vi "ROI selection.vi"(2 "ROI":T1={"Far Field  Row"=72, "Far Field Col"=185, "Far Field outer radius"=62, "Far Field inner radius"=62}, 3 "Far Field pixels":T2, 4 "Near Field pixels":T3) -> (0 "Far Field ROI":T2, 1 "Near Field ROI":T3)   [LabVIEW 2020]
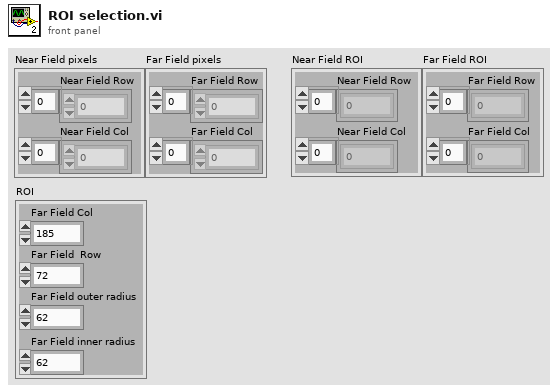
[diagram p1: front panel]
types:
  T1 = cluster{"Far Field  Row":i32, "Far Field Col":i32, "Far Field outer radius":i32, "Far Field inner radius":i32}
  T2 = cluster{"Far Field Row":dbl[], "Far Field Col":dbl[]}
  T3 = cluster{"Near Field Row":dbl[], "Near Field Col":dbl[]}
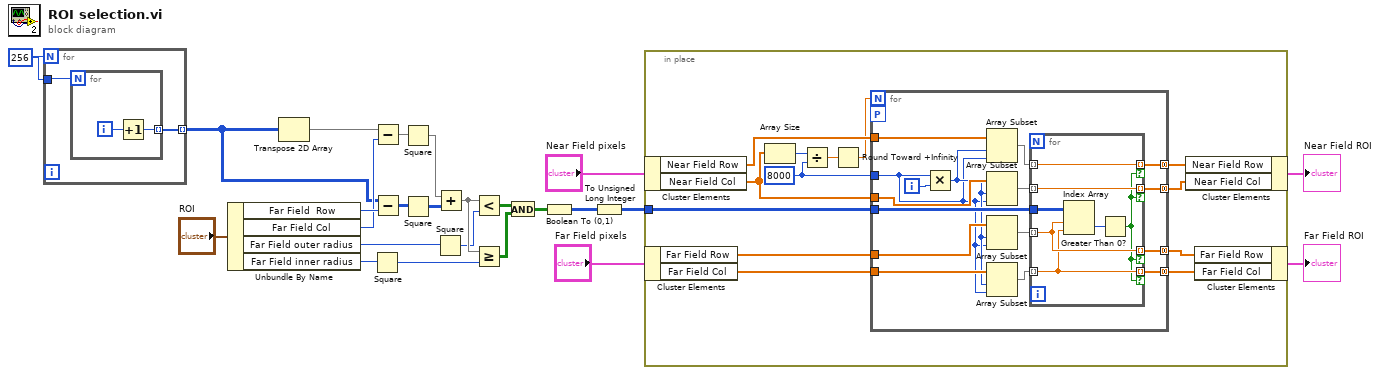
[diagram p0: block diagram]
diagram:
  w24 = 256
  n1 = for {
    N: w24 -> [_]
    tunnel: w24 -> [w26]
    tunnel: [w25] -> w15 mode=indexing
    n2 = for {
      N: w26 -> [_]
      tunnel: [w28] -> w25 mode=indexing
      i -> [w27]
      n3 = Increment(x=w27) -> (x+1=w28:i32)
    }
  }
  n4 = Unbundle By Name("ROI") -> ("Far Field  Row"=w18:i32, "Far Field Col"=w17:i32, "Far Field outer radius"=w5:i32, "Far Field inner radius"=w1:i32)
  n5 = Transpose 2D Array(2D array=w15) -> (transposed array=w16:i32[][])
  n6 = Square(x=w1) -> (x^2=w4:i32)
  n7 = Subtract(x=w16, y=w17) -> (x-y=w23:i32[][])
  n8 = Subtract(x=w15, y=w18) -> (x-y=w22:i32[][])
  n9 = Square(x=w23) -> (x^2=w21:i32[][])
  n10 = Square(x=w22) -> (x^2=w20:i32[][])
  n11 = Square(x=w5) -> (x^2=w6:i32)
  n12 = Add(x=w21, y=w20) -> (x+y=w7:i32[][])
  n13 = Less?(x=w7, y=w6) -> (x < y?=w9:bool[][])
  n14 = Greater Or Equal?(x=w7, y=w4) -> (x >= y?=w8:bool[][])
  n15 = And(x=w9, y=w8) -> (x .and. y?=w3:bool[][])
  n16 = Boolean To (0,1)(Boolean=w3) -> (0, 1=w19:i16[][])
  n17 = To Unsigned Long Integer(number=w19) -> (unsigned 32bit integer=w12:u32[][])
  n18 = in-place {
    in-place-border: w12 -> [w41]
    w32 = 8000
    n19 = in-place-cluster #1("Near Field pixels") -> ("Near Field Row"=w38:dbl[], "Near Field Col"=w33:dbl[])
    n20 = in-place-cluster #2("Far Field pixels") -> ("Far Field Row"=w40:dbl[], "Far Field Col"=w39:dbl[])
    n21 = Array Size(array=w33) -> (size(s)=w34:i32)
    n22 = Divide(x=w34, y=w32) -> (x/y=w30:dbl)
    n23 = Round Toward +Infinity(x=w30) -> (ceil(x): smallest int >= x=w29:dbl)
    n24 = for {
      N: w29 -> [_]
      tunnel: w38 -> [w56]
      tunnel: w33 -> [w53]
      tunnel: w40 -> [w51]
      tunnel: w39 -> [w49]
      tunnel: w41 -> [w57]
      tunnel: [w46] -> w37 mode=concatenating
      tunnel: [w45] -> w36 mode=concatenating
      tunnel: [w44] -> w35 mode=concatenating
      tunnel: [w43] -> w31 mode=concatenating
      tunnel: w32 -> [w42]
      workers-P: _ -> [_]
      i -> [w54]
      n25 = Multiply(x=w42, y=w54) -> (x*y=w47:i32)
      n26 = Array Subset(array=w56, index=w47, length=w42) -> (w55:dbl[])
      n27 = Array Subset(array=w53, index=w47, length=w42) -> (w52:dbl[])
      n28 = Array Subset(array=w51, index=w47, length=w42) -> (w50:dbl[])
      n29 = Array Subset(array=w49, index=w47, length=w42) -> (w48:dbl[])
      n30 = for {
        tunnel: w55 -> [w63] mode=indexing
        tunnel: w52 -> [w62] mode=indexing
        tunnel: w50 -> [w61] mode=indexing
        tunnel: w48 -> [w60] mode=indexing
        tunnel: w57 -> [w64]
        tunnel: [w63] -> w46 mode=indexing if=w58
        tunnel: [w62] -> w45 mode=indexing if=w58
        tunnel: [w61] -> w44 mode=indexing if=w58
        tunnel: [w60] -> w43 mode=indexing if=w58
        n31 = Index Array(array=w64, index (row)=w61, index (col)=w60) -> (element=w59:u32)
        n32 = Greater Than 0?(x=w59) -> (x > 0?=w58:bool)
      }
    }
    n33 = in-place-cluster #1("Near Field Row"=w37, "Near Field Col"=w36) -> (→"Near Field ROI":T3)
    n34 = in-place-cluster #2("Far Field Row"=w35, "Far Field Col"=w31) -> (→"Far Field ROI":T2)
  }
